vi "ChannelList_Attributes_GetProperty.vi"(8 "error in (no error)":errorcluster, 9 "Property Name":string, 10 "Channel ID":string, 11 "OXY_SCPI Reseource In":refnum<visa-resource-name>) -> (0 "error out":errorcluster, 1 "communication_data":T1, 2 "Property Value":string, 3 "OXY_SCPI Reseource Out":refnum<visa-resource-name>)   [LabVIEW 2020, in "OXYGEN_Datastream.lvlib"]
doc: "Queries a specific property (config-item) of a given channel."
uses:
  OXYGEN_Datastream.lvlib
  TypeDefs/Cluster_RawCommData.ctl
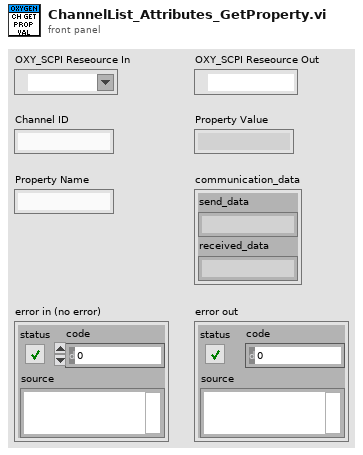
[diagram p1: front panel]
types:
  T1 = typedef "OXYGEN_Datastream.lvlib/Cluster_RawCommData.ctl" = cluster{"send_data":string, "received_data":string}
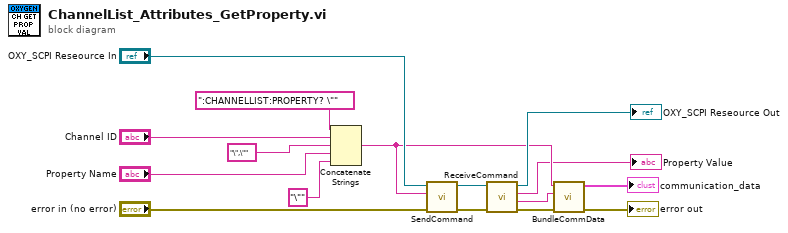
[diagram p0: block diagram]
diagram:
  n1 = Concatenate Strings(":CHANNELLIST:PROPERTY? \"", "Channel ID", "\",\"", "Property Name", "\"" ("string")) -> (w4:string)
  n2 = call "SendCommand.vi"("error in (no error)"="error in (no error)", "String to Send"=w4, "OXY_SCPI Reseource In"="OXY_SCPI Reseource In") -> ("error out"=w16:errorcluster, "OXY_SCPI Reseource Out"=w15:refnum<visa-resource-name>)  [unwired: 7 in]
  n3 = call "ReceiveCommand.vi"("error in (no error)"=w16, "OXY_SCPI Reseource In"=w15) -> ("error out"=w11:errorcluster, "received Data with Header"=w9:string, "received Data"=→"Property Value":string, "OXY_SCPI Reseource Out"=→"OXY_SCPI Reseource Out":refnum<visa-resource-name>)  [unwired: 6 in]
  n4 = call "BundleCommData.vi"("error in (no error)"=w11, "received_data"=w9, "send_data"=w4) -> ("error out"=→"error out":errorcluster, "communication_data"=→"communication_data":T1)  [unwired: 7 in]
